vi "DAQmx.44xx.Get Terminal Configuration.vi"(8 "error in (no error)":errorcluster, 9 "Channel in":tag, 11 "terminal configuration in":i32) -> (0 "error out":errorcluster, 3 "terminal configuration out":i32)   [LabVIEW 2019, in "DAQmx.lvclass"]
uses:
  DAQmx.lvclass
  typedefs/DAQ.Config.Device Type--enum.ctl
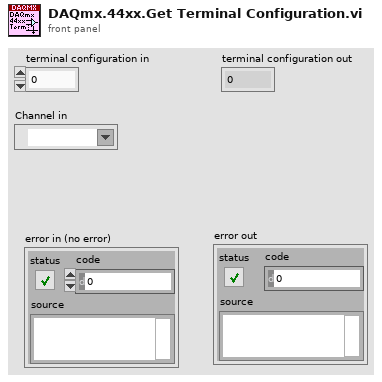
[diagram p1: front panel]
types:
  T1 = typedef "DAQmx.lvclass/DAQ.Config.Device Type--enum.ctl" = enum16{"None", "USB-4431", "PXI-446x"}
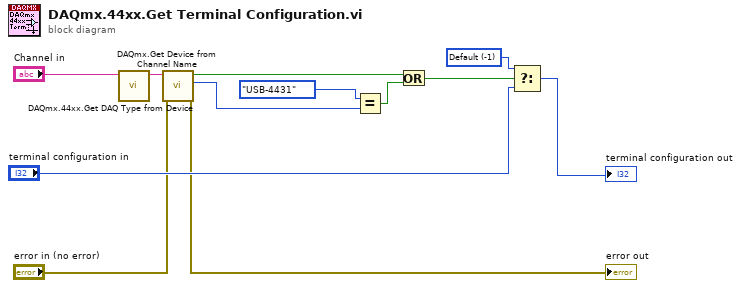
[diagram p0: block diagram]
diagram:
  w7 = -1 items=["Default"=-1, "RSE"=10083, "Differential"=10106, "Pseudodifferential"=12529] ("output terminal configuration")
  n1 = call "DAQmx.Get Device from Channel Name.vi"("Channel"="Channel in") -> ("Device"=w6:tag)  [unwired: 10 in]
  n2 = call "DAQmx.44xx.Get DAQ Type from Device.vi"("error in (no error)"="error in (no error)", "DAQmx Device Name"=w6) -> ("error out"=→"error out":errorcluster, "DAQ Type"=w2:T1, "DevIsSimulated"=w9:bool)  [unwired: 7 in]
  n3 = Equal?(x=DAQ.Config.Device_Type--enum."USB-4431" ("DAQ Type"), y=w2) -> (x = y?=w8:bool)
  n4 = Or(x=w9, y=w8) -> (x .or. y?=w10:bool)
  n5 = Select(t=w7, s=w10, f="terminal configuration in") -> (s? t:f=→"terminal configuration out":i32)
